vi "RTC_reader.vi"() -> ()   [LabVIEW 2015]
uses:
  <vilib>/Instr/_visa.llb/VISA Configure Serial Port (Instr).vi
panel:
  out "Numeric Indicator":u64
  out "String":string
  in  "VISA resource name":refnum<visa-resource-name>
  out "MMSB2":u8 format="%x"
  out "MSB":u8 format="%x"
  in  "stop":bool
  out "LSB":u8 format="%x"
  out "MMSB1":u8 format="%x"
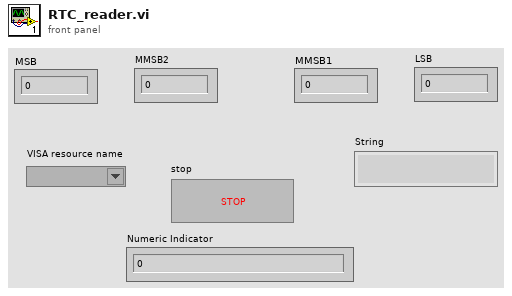
[diagram p1: front panel]
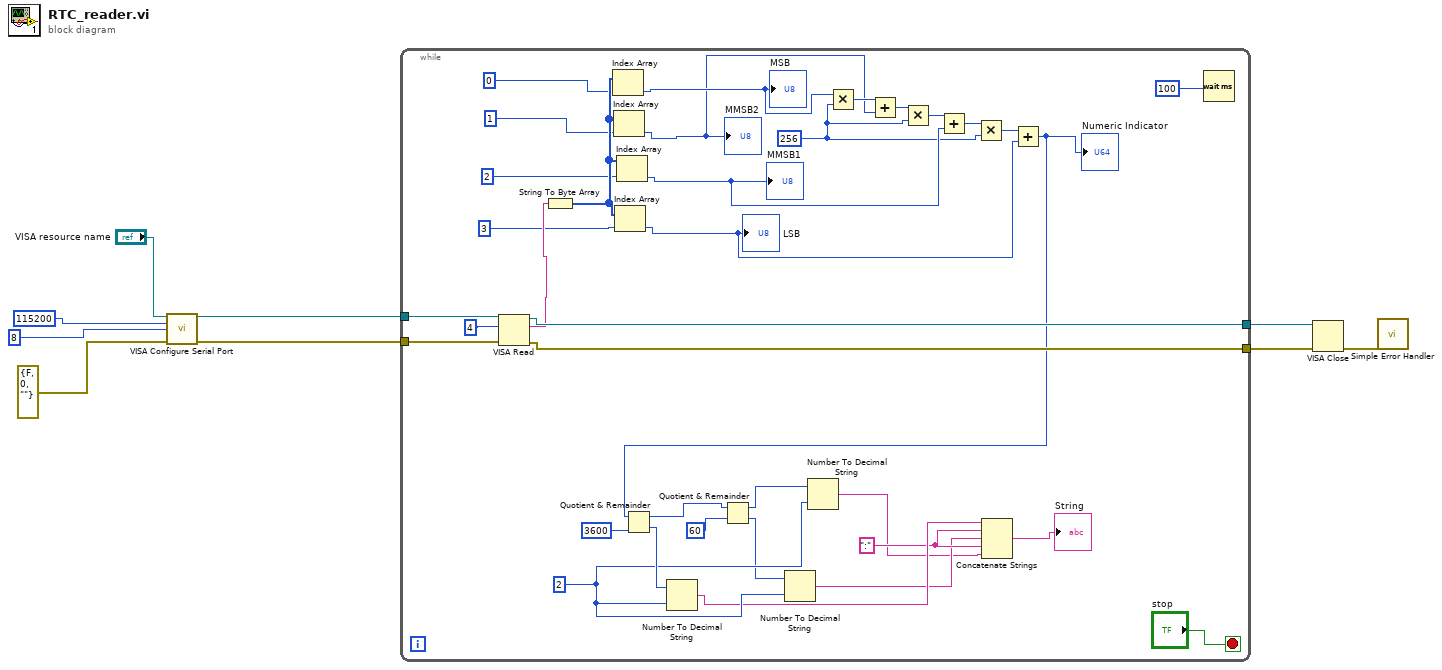
[diagram p0: block diagram]
diagram:
  n1 = call-poly "VISA Configure Serial Port"("VISA resource name"="VISA resource name", "baud rate (9600)"=115200, "data bits (8)"=8, "error in (no error)"=errorcluster {"status"=FALSE, "code"=0, "source"=""} ("error constant")) -> ("VISA resource name out"=w6:refnum<visa-resource-name>, "error out"=w5:errorcluster)  [unwired: 10 in]
  n2 = while {
    tunnel: w6 -> [w43]
    tunnel: w5 -> [w42]
    tunnel: [w41] -> w4
    tunnel: [w40] -> w3
    stop <- "stop" stop-if-true
    w13 = ":"
    w17 = 2
    w25 = 256
    n3 = VISA Read(VISA resource name=w43, byte count=4, error in (no error)=w42) -> (VISA resource name out=w41:refnum<visa-resource-name>, read buffer=w38:string, error out=w40:errorcluster)  [unwired: 1 out]
    n4 = String To Byte Array(string=w38) -> (unsigned byte array=w37:u8[])
    n5 = Index Array(array=w37, index=0) -> (element=w32:u8)
    "MSB" <- w32
    n6 = Index Array(array=w37, index=1) -> (element=w30:u8)
    "MMSB2" <- w30
    n7 = Index Array(array=w37, index=3) -> (element=w23:u8)
    "LSB" <- w23
    n8 = Index Array(array=w37, index=2) -> (element=w27:u8)
    "MMSB1" <- w27
    n9 = Multiply(x=w32, y=w25) -> (x*y=w31:i32)
    n10 = Add(x=w31, y=w30) -> (x+y=w29:i32)
    n11 = Multiply(x=w29, y=w25) -> (x*y=w28:i32)
    n12 = Add(x=w28, y=w27) -> (x+y=w26:i32)
    n13 = Multiply(x=w26, y=w25) -> (x*y=w24:i32)
    n14 = Add(x=w24, y=w23) -> (x+y=w22:i32)
    "Numeric Indicator" <- w22
    n15 = Quotient & Remainder(x=w22, y=3600) -> (x-y*floor(x/y)=w20:i32, floor(x/y)=w18:i32)
    n16 = Number To Decimal String(number=w18, width (-)=w17) -> (decimal integer string=w14:string)
    n17 = Quotient & Remainder(x=w20, y=60) -> (x-y*floor(x/y)=w15:i32, floor(x/y)=w16:i32)
    n18 = Number To Decimal String(number=w16, width (-)=w17) -> (decimal integer string=w12:string)
    n19 = Number To Decimal String(number=w15, width (-)=w17) -> (decimal integer string=w11:string)
    n20 = Concatenate Strings(w14, w13, w12, w13, w11) -> (→"String":string)
    n21 = Wait (ms)(milliseconds to wait=100) -> ()  [unwired: 1 out]
  }
  n22 = VISA Close(VISA resource name=w4, error in (no error)=w3) -> (error out=w2:errorcluster)
  n23 = call <vilib>:"Simple Error Handler.vi"("error in (no error)"=w2) -> ()  [unwired: 4 in, 5 out]
